vi "_Build Create.vi"(8 "error in (no error)":errorcluster, 9 "tableName":string, 10 "DynamicParameters in":refnum<class "DynamicParameters.lvclass">, 11 "PostgresqlConnection in":refnum<class "DBC.lvclass">) -> (0 "error out":errorcluster, 1 "QueryString Out":string, 2 "Insert Exec Out":string, 3 "PostgresqlConnection out":refnum<class "DBC.lvclass">)   [LabVIEW 2020, in "ORM_DBC_Npgsql.lvlib" / "DBC.lvclass"]
uses:
  DBC.lvclass
  C:/Program Files/National Instruments/LabVIEW 2024/vi.lib/Viviota/shared/ORM.lvlibp/ORM/DbConnection/DbConnection.lvclass
  <vilib>/Viviota/shared/ORM.lvlibp/ORM/DynamicParameters/DynamicParameters.lvclass
  <vilib>/Viviota/shared/ORM.lvlibp/ORM/DbConnection/Read ColumnNameFormat.vi
  <vilib>/Viviota/shared/ORM.lvlibp/ORM/DbConnection/Read LastIdentityQuery.vi
  <vilib>/Viviota/shared/ORM.lvlibp/ORM/DynamicParameters/Read ParameterNames.vi
  <vilib>/Viviota/shared/ORM.lvlibp/ORM/DynamicParameters/Read FieldNames.vi
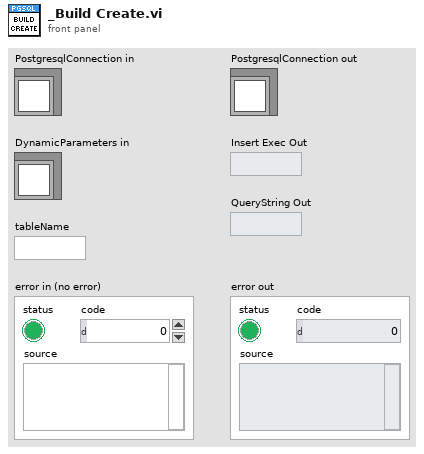
[diagram p1: front panel]
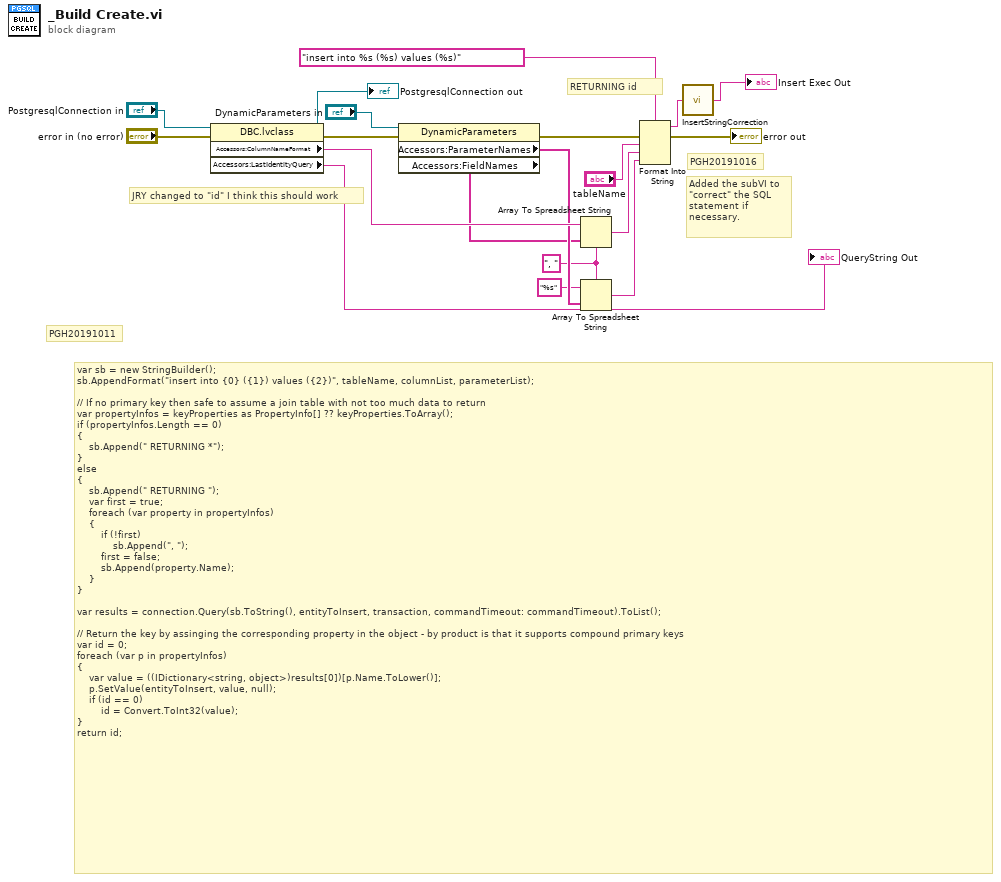
[diagram p0: block diagram]
diagram:
  w15 = ", " ("delimiter (Tab)")
  # "RETURNING id"
  # "Added the subVI to\n\"correct\" the SQL \nstatement if\nnecessary."
  # "PGH20191016"
  # "PGH20191011"
  # "var sb = new StringBuilder();\nsb.AppendFormat(\"insert into {0} ({1}) values ({2})\", tableName, columnList, parameterList);\n\n// If no primary key then safe to assume a join table with not too much data to return\nvar propertyInfos = keyProperties as PropertyInfo[] ?? keyProperties.ToArray();\nif (propertyInfos.Length == 0)\n{\n    sb.Append(\" RETURNING *\");\n}\nelse\n{\n    sb.Append(\" RETURNING \");\n    var first = true;\n    foreach (var property in propertyInfos)\n    {\n        if (!first)\n            sb.Append(\", \");\n        first = false;\n        sb.Append(property.Name);\n    }\n}\n\nvar results = connection.Query(sb.ToString(), entityToInsert, transaction, commandTimeout: commandTimeout).ToList();\n\n// Return the key by assinging the corresponding property in the object - by product is that it supports compound primary keys\nvar id = 0;\nforeach (var p in propertyInfos)\n{\n    var value = ((IDictionary<string, object>)results[0])[p.Name.ToLower()];\n    p.SetValue(entityToInsert, value, null);\n    if (id == 0)\n        id = Convert.ToInt32(value);\n}\nreturn id;"
  # "JRY changed to \"id\" I think this should work"
  n1 = property class="DBC.lvclass"(reference="PostgresqlConnection in", error in="error in (no error)") -> (reference out=→"PostgresqlConnection out":refnum<class "DBC.lvclass">, error out=w7:errorcluster, "Accessors:ColumnNameFormat"=w18:string, "Accessors:LastIdentityQuery"=→"QueryString Out":string)
  n2 = property class="DynamicParameters"(reference="DynamicParameters in", error in=w7) -> (error out=w6:errorcluster, "Accessors:ParameterNames"=w16:string[], "Accessors:FieldNames"=w2:string[])  [unwired: 1 out]
  n3 = Array To Spreadsheet String(delimiter (Tab)=w15, array=w2, 3:w18) -> (spreadsheet string=w12:string)
  n4 = Array To Spreadsheet String(delimiter (Tab)=w15, array=w16, 3:"%s" ("format string")) -> (spreadsheet string=w17:string)
  n5 = Format Into String(format string="insert into %s (%s) values (%s)", error in=w6, "tableName", w12, w17) -> (resulting string=w19:string, error out=→"error out":errorcluster)  [unwired: 1 in]
  n6 = call "InsertStringCorrection.vi"("SQL string"=w19) -> ("SQL String Out"=→"Insert Exec Out":string)  [unwired: 4 in]
